vi "CheckStepNameLength.vi"(8 "error in (no error)":errorcluster, 9 "RuleConfiguration In":refnum<k7>, 10 "Step In":refnum<k7>, 11 "AnalysisContext In":refnum<k7>) -> (0 "error out":errorcluster, 1 "RuleConfiguration Out":refnum<k7>, 2 "Step Out":refnum<k7>, 3 "AnalysisContext Out":refnum<k7>)   [LabVIEW 2011]
uses:
  StepNameLengthRuleConstants.vi
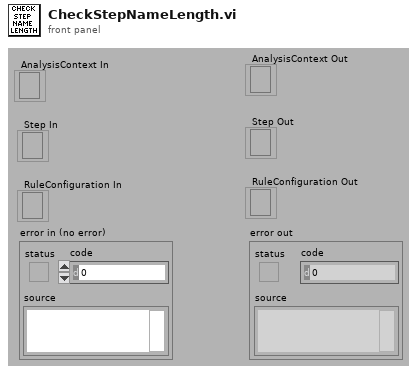
[diagram p1: front panel]
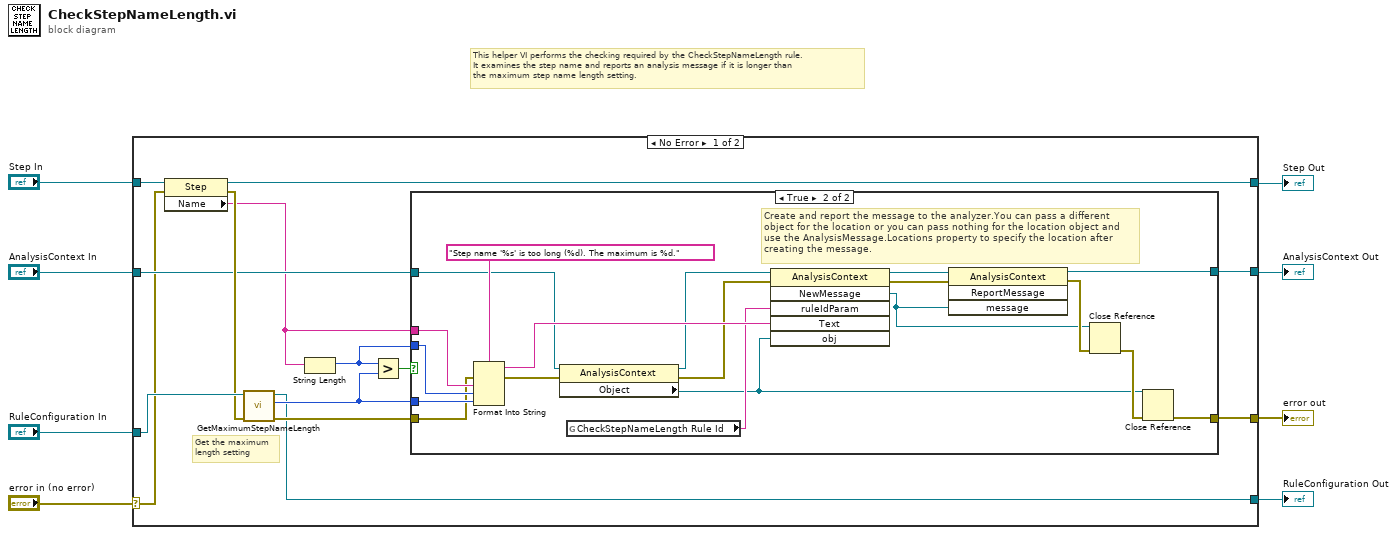
[diagram p0: block diagram]
diagram:
  # "This helper VI performs the checking required by the CheckStepNameLength rule.\nIt examines the step name and reports an analysis message if it is longer than\nthe maximum step name length setting."
  n1 = case shown="No Error" "error in (no error)" {
    selector: "error in (no error)" -> [w9 w47]
    tunnel: "Step In" -> [w22 w46]
    tunnel: "RuleConfiguration In" -> [w21 w44]
    tunnel: "AnalysisContext In" -> [w18 w45]
    tunnel: [w13 w47] -> w5
    tunnel: [w12 w45] -> w4
    tunnel: [w11 w44] -> w3
    tunnel: [w10 w46] -> w2
    frame No Error {
      # "Get the maximum\nlength setting"
      n2 = property class="Step"(reference=w22, error in=w9) -> (reference out=w10:refnum<k7>, error out=w19:errorcluster, "Name"=w17:string)
      n3 = call "GetMaximumStepNameLength.vi"("error in (no error)"=w19, "RuleConfiguration in"=w21) -> ("error out"=w14:errorcluster, "Maximum Step Name Length"=w15:i32, "RuleConfiguration out"=w11:refnum<k7>)  [unwired: 3 out]
      n4 = String Length(string=w17) -> (length=w16:i32)
      n5 = Greater?(x=w16, y=w15) -> (0:w20:bool)
      n6 = case shown="True" w20 {
        tunnel: w18 -> [w23 w36]
        tunnel: w17 -> [_ w42]
        tunnel: w16 -> [_ w41]
        tunnel: w15 -> [_ w40]
        tunnel: w14 -> [w24 w39]
        tunnel: [w23 w30] -> w12
        tunnel: [w24 w27] -> w13
        frame False {
        }
        frame True {
          # "Create and report the message to the analyzer.You can pass a different object for the location or you can pass nothing for the location object and use the AnalysisMessage.Locations property to specify the location after creating the message."
          n7 = Format Into String(format string="Step name '%s' is too long (%d). The maximum is %d.", error in=w39, w42, w41, w40) -> (resulting string=w38:string, error out=w31:errorcluster)  [unwired: 1 in]
          n8 = property class="AnalysisContext"(reference=w36, error in=w31) -> (reference out=w35:refnum<k7>, error out=w37:errorcluster, "Object"=w25:refnum<k7>)
          n9 = global read "StepNameLengthRuleConstants.vi" "CheckStepNameLength Rule Id"() -> (w34:string)
          n10 = invoke class="AnalysisContext" method="NewMessage"(reference=w35, error in=w37, "ruleIdParam"=w34, "Text"=w38, "obj"=w25) -> (reference out=w33:refnum<k7>, error out=w32:errorcluster, "NewMessage"=w26:refnum<k7>)  [unwired: 1 in, 3 out]
          n11 = invoke class="AnalysisContext" method="ReportMessage"(reference=w33, error in=w32, "message"=w26) -> (reference out=w30:refnum<k7>, error out=w29:errorcluster)  [unwired: 1 in, 2 out]
          n12 = Close Reference(reference=w26, error in (no error)=w29) -> (error out=w28:errorcluster)
          n13 = Close Reference(reference=w25, error in (no error)=w28) -> (error out=w27:errorcluster)
        }
      }
    }
    frame Error {
    }
  }
  "error out" <- w5
  "AnalysisContext Out" <- w4
  "Step Out" <- w2
  "RuleConfiguration Out" <- w3
